vi "Configure Hardware.vi"(8 "error in (no error)":errorcluster, 10 "Active_Profile":T1, 11 "Hardware Resources in":T2) -> (0 "error out":errorcluster, 3 "Hardware Resources out":T2)   [LabVIEW 2026, in "Acquisition.lvlib"]
doc: "Configure the hardware."
uses:
  Acquisition.lvlib
  Controls/Hardware Configuration.ctl
  Controls/Vibration_Profile.ctl
  <vilib>/DAQmx/configure/timing.llb/DAQmx Timing (Sample Clock).vi
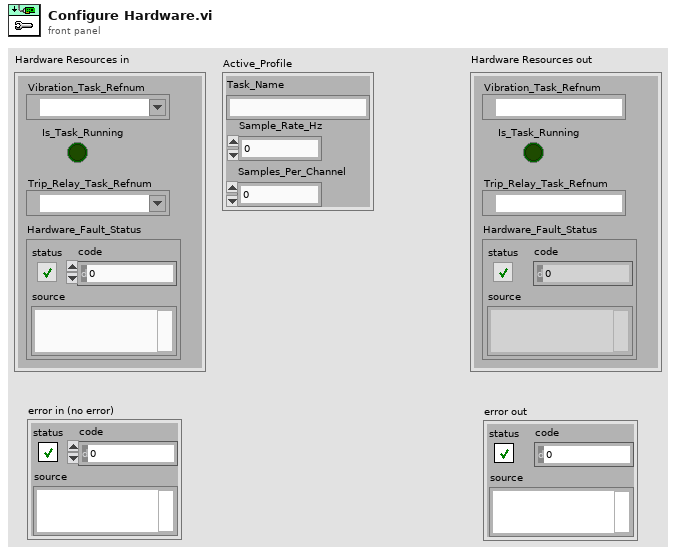
[diagram p1: front panel]
types:
  T1 = typedef "Vibration_Profile.ctl" = cluster{"Task_Name":string, "Sample_Rate_Hz":dbl, "Samples_Per_Channel":i32}
  T2 = typedef "Acquisition.lvlib/Hardware Configuration.ctl" = cluster{"Vibration_Task_Refnum":refnum<k21>, "Is_Task_Running":bool, "Hardware_Fault_Status":errorcluster, "Trip_Relay_Task_Refnum":refnum<k21>}
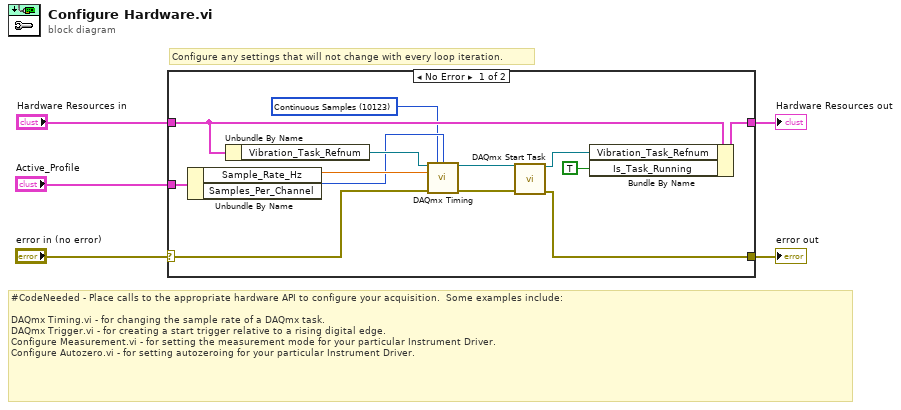
[diagram p0: block diagram]
diagram:
  # "Configure any settings that will not change with every loop iteration."
  # "#CodeNeeded - Place calls to the appropriate hardware API to configure your acquisition.  Some examples include:\n\nDAQmx Timing.vi - for changing the sample rate of a DAQmx task.\nDAQmx Trigger.vi - for creating a start trigger relative to a rising digital edge.\nConfigure Measurement.vi - for setting the measurement mode for your particular Instrument Driver.\nConfigure Autozero.vi - for setting autozeroing for your particular Instrument Driver."
  n1 = case shown="No Error" "error in (no error)" {
    selector: "error in (no error)" -> [w15 w19]
    tunnel: [w11 w19] -> w4
    tunnel: "Hardware Resources in" -> [w17 w20]
    tunnel: [w18 w20] -> w2
    tunnel: "Active_Profile" -> [w14 _]
    frame No Error {
      w6 = 10123 items=["Finite Samples"=10178, "Continuous Samples"=10123, "Hardware Timed Single Point"=12522] ("sample mode")
      n2 = Unbundle By Name(w14) -> ("Sample_Rate_Hz"=w13:dbl, "Samples_Per_Channel"=w7:i32)
      n3 = Unbundle By Name(w17) -> ("Vibration_Task_Refnum"=w16:refnum<k21>)
      n4 = call-poly <vilib>:"DAQmx Timing.vi"("task/channels in"=w16, "sample mode"=w6, "samples per channel"=w7, "rate"=w13, "error in"=w15) -> ("task out"=w10:refnum<k21>, "error out"=w12:errorcluster)  [unwired: 9 in]
      n5 = call <vilib>:"DAQmx Start Task.vi"("task/channels in"=w10, "error in"=w12) -> ("task out"=w9:refnum<k21>, "error out"=w11:errorcluster)  [unwired: 12 in]
      n6 = Bundle By Name(cluster=w17, "Vibration_Task_Refnum"=w9, "Is_Task_Running"=TRUE) -> (w18:T2)
    }
    frame Error {
    }
  }
  "Hardware Resources out" <- w2
  "error out" <- w4
